vi "test udp++2.vi"() -> ()   [LabVIEW 2017]
uses:
  <vilib>/Platform/TimedLoop/XDataNode/timing_clust.ctl
  <vilib>/Platform/TimedLoop/XDataNode/nitl_modes.ctl
  <vilib>/Platform/TimedLoop/XDataNode/wakeup.ctl
  <vilib>/Platform/TimedLoop/XDataNode/XDataNode.xnode
  <vilib>/Platform/TimedLoop/XDataNode/XDNodeRunTimeDep.lvlib
  UDP++.lvlib
panel:
  in  "stop":bool
  out "sumcheck":dbl[](array[numeric])
  out "Validation send":dbl[](array[numeric])
  in  "Numeric":i32=1000
  out "Array":dbl[](array[numeric])
  out "接收控制指令":dbl[](array[numeric])
  out "wifi_KongZ":bool
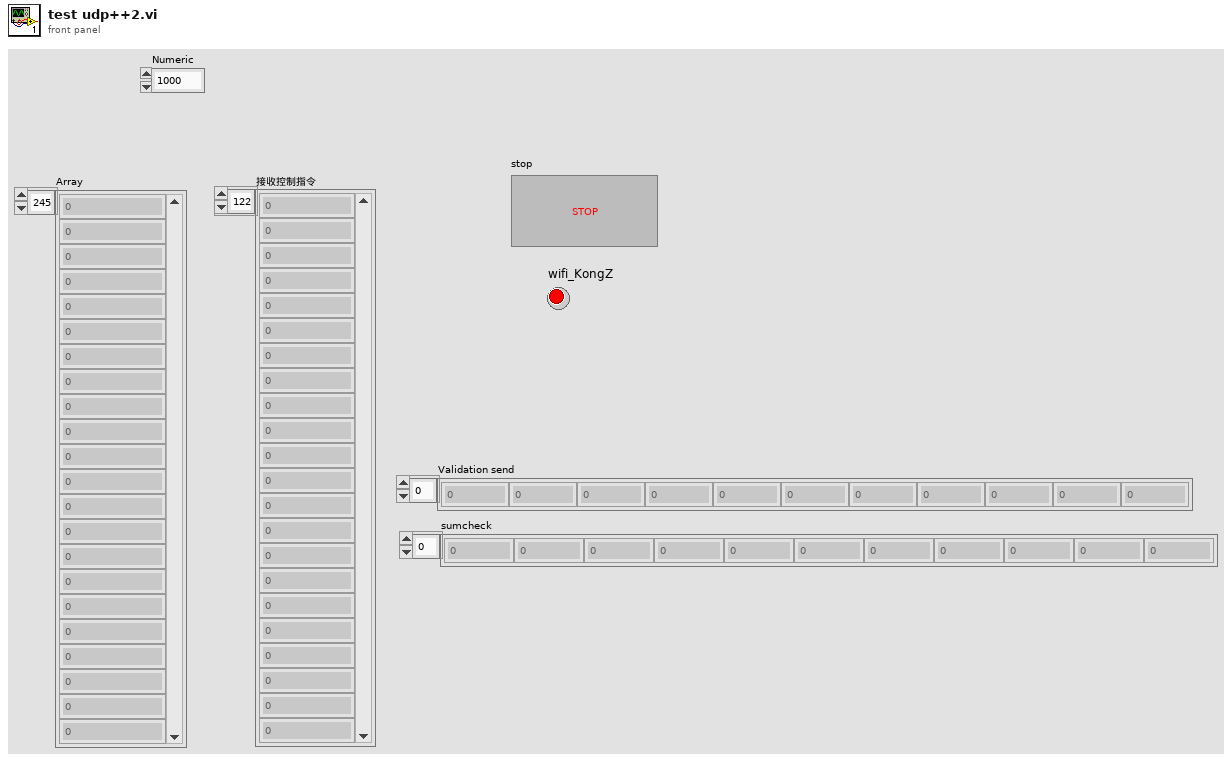
[diagram p1: front panel]
types:
  T1 = cluster{"本地IP":string, "本地端口":u16, "远程IP":string, "远程端口":u16}
  T2 = typedef "XDNodeRunTimeDep.lvlib/timing_clust.ctl" = cluster{"Expected End [f-1]":u64, "Actual End [f-1]":u64, "Finished Late? [f-1]":bool, "Expected End [i-1]":u64, "Actual End [i-1]":u64, "Finished Late? [i-1]":bool, "Expected Start [i]":u64, "Actual Start [i]":u64, "Expected Start [f]":u64, "Actual Start [f]":u64, "Source Name":string, "Structure Name":string, "Period":i64, "Deadline":i64, "Offset":i64, "Start":i64, "Priority":i32, "Timeout":i32, "Mode":T3, "Wakeup Reason":T4, "Error":errorcluster, "Source Type":string, "Secondary Source Type":string, "Global End Time":u64, "Global Start Time":u64, "Frame Duration":u64, "Iteration Duration":u64, "Assigned CPU":i32, "I/O Scan Engine Mode":u32}
  T3 = typedef "XDNodeRunTimeDep.lvlib/nitl_modes.ctl" = enum32{"No Change", "Process missed periods, maintain original phase", "Discard missed periods, maintain original phase", "Process missed periods, ignore original phase", "Discard missed periods, ignore original phase"}
  T4 = typedef "XDNodeRunTimeDep.lvlib/wakeup.ctl" = enum32{"Normal", "Aborted", "Asynchronous wakeup", "Timing source error", "Timed loop error", "Timeout"}
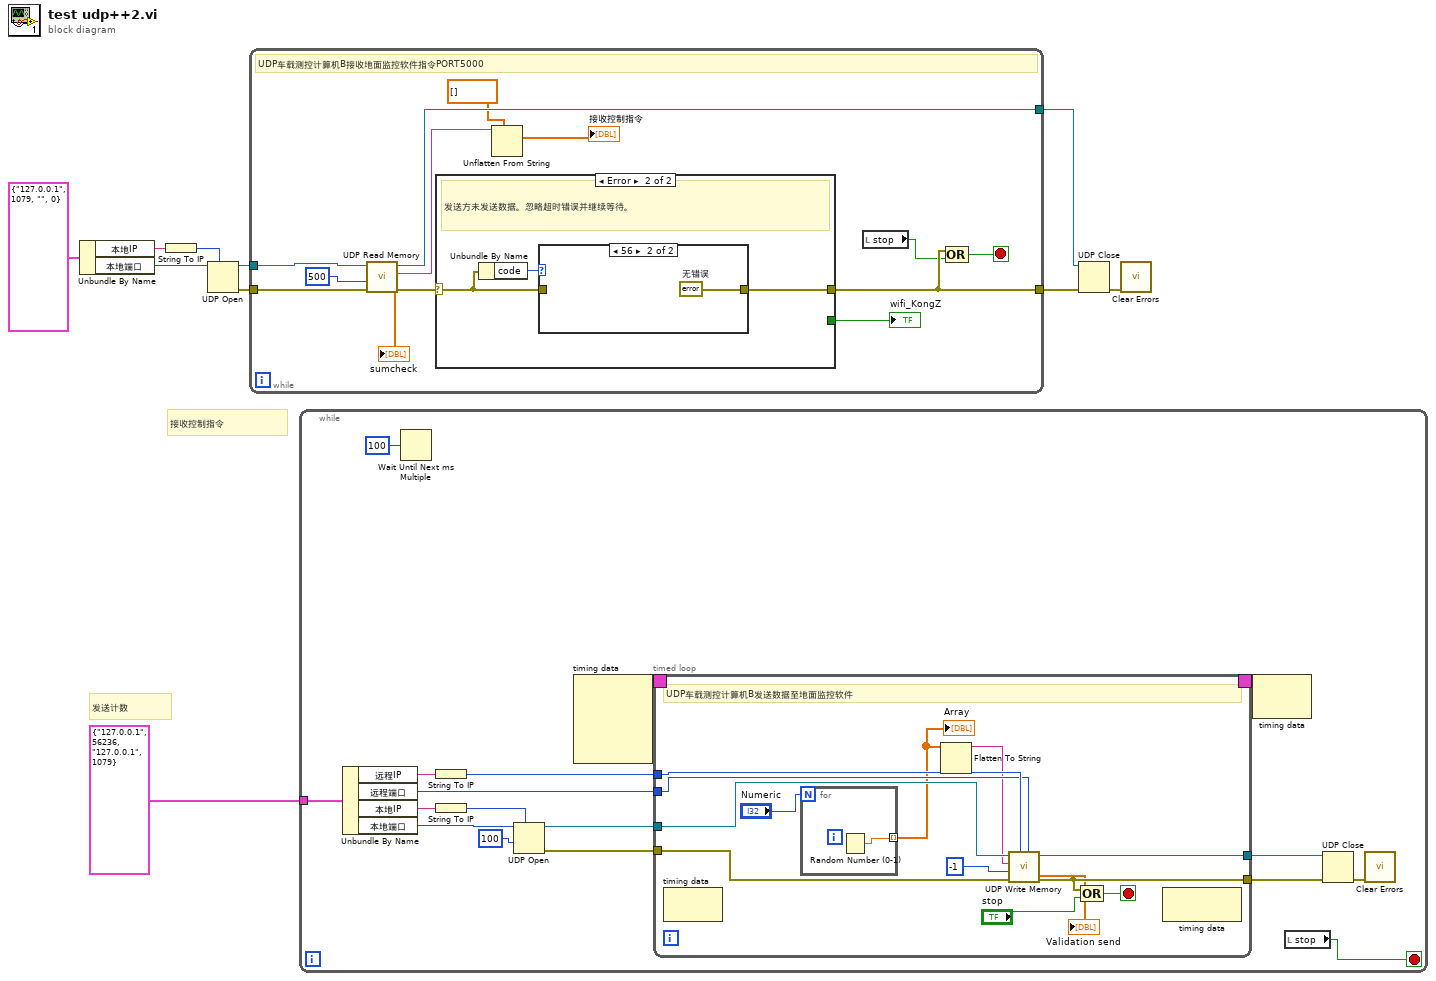
[diagram p0: block diagram]
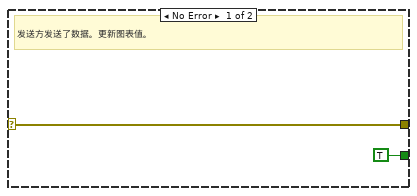
[diagram p2: hidden frame]
diagram:
  # "发送计数"
  # "接收控制指令"
  n1 = Unbundle By Name(T1 {"本地IP"="127.0.0.1", "本地端口"=1079, "远程IP"="", "远程端口"=0} ("UDP配置")) -> ("本地IP"=w3:string, "本地端口"=w2:u16)
  n2 = String To IP(1:w3) -> (0:w10:u32)
  n3 = UDP Open(7:w10, 11:w2) -> (port=w9:refnum<k16>, 0:w8:errorcluster)  [unwired: 3 in, 1 out]
  n4 = while {
    tunnel: w9 -> [w23]
    tunnel: [w21] -> w6
    tunnel: w8 -> [w22]
    tunnel: [w20] -> w7
    stop <- w19 stop-if-true
    # "UDP车载测控计算机B接收地面监控软件指令PORT5000"
    n5 = call "UDP Read Memory.vi"("error in (no error)"=w22, "超时毫秒(25000)"=500, "UDP Network Connection in"=w23) -> ("error out"=w17:errorcluster, "String"=w15:string, "UDP Network Connection out"=w21:refnum<k16>, "checksum"=→"sumcheck":dbl[])  [unwired: 5 in]
    n6 = case shown="Error" w17 {
      selector: w17 -> [w25 w27]
      tunnel: [w25 w26] -> w20
      tunnel: [TRUE ("wifi_KongZ") _] -> w18
      frame No Error {
        # "发送方发送了数据。更新图表值。"
      }
      frame Error {
        # "发送方未发送数据。忽略超时错误并继续等待。"
        n7 = Unbundle By Name(w27) -> ("code"=w28:i32)
        n8 = case shown="56" w28 {
          tunnel: w27 -> [w29 _]
          tunnel: [w29 w30] -> w26
          frame Default {
          }
          frame 56 {
            w30 = errorcluster {"status"=FALSE, "code"=0, "source"=""}  # 无错误
          }
        }
      }
    }
    "wifi_KongZ" <- w18
    n9 = Unflatten From String(type=dbl[] [] ("接收控制指令"), binary string=w15) -> (value=→"接收控制指令":dbl[])  [unwired: 3 in, 2 out]
    n10 = local read "stop"() -> (w11:bool)
    n11 = Compound Arithmetic op=OR ("复合运算")(w20, w11) -> (w19:bool)
  }
  n12 = while {
    tunnel: T1 {"本地IP"="127.0.0.1", "本地端口"=56236, "远程IP"="127.0.0.1", "远程端口"=1079} ("UDP配置") -> [w36]
    stop <- w31 stop-if-true
    n13 = Unbundle By Name(w36) -> ("远程IP"=w33:string, "远程端口"=w32:u16, "本地IP"=w34:string, "本地端口"=w35:u16)
    n14 = Wait Until Next ms Multiple(millisecond multiple=u32 100 ("毫秒倍数")) -> ()  [unwired: 1 out]
    n15 = String To IP(1:w33) -> (0:w41:u32)
    n16 = String To IP(1:w34) -> (0:w43:u32)
    n17 = UDP Open(7:w43, 9:100 ("超时毫秒(25000)"), 11:w35) -> (port=w45:refnum<k16>, 0:w44:errorcluster)  [unwired: 2 in, 1 out]
    n18 = node-c288() -> (w47:T2)  [unwired: 4 in]
    n19 = timed-loop {
      tunnel: [w57] -> w39
      tunnel: w45 -> [w60]
      tunnel: w44 -> [w58]
      tunnel: [w59] -> w38
      tunnel: w32 -> [w53]
      timing: w47 -> [_]
      timing-out: [_] -> w46
      tunnel: w41 -> [w54]
      stop <- w56 stop-if-true
      # "UDP车载测控计算机B发送数据至地面监控软件"
      n20 = node-c288() -> ()  [unwired: 1 in, 1 out]
      n21 = for {
        N: "Numeric" -> [_]
        tunnel: [w61] -> w51 mode=indexing
        n22 = Random Number (0-1)() -> (number: 0 to 1=w61:dbl)
      }
      "Array" <- w51
      n23 = Flatten To String(anything=w51) -> (data string=w50:string)  [unwired: 3 in, 2 out]
      n24 = call "UDP Write Memory.vi"("port or service name"=w53, "address"=w54, "error in (no error)"=w58, "超时毫秒(25000)"=-1, "String"=w50, "UDP Network Connection in"=w60) -> ("error out"=w57:errorcluster, "UDP Network Connection out"=w59:refnum<k16>, "checksum"=→"Validation send":dbl[])  [unwired: 3 in]
      n25 = Compound Arithmetic op=OR ("复合运算")(w57, "stop") -> (w56:bool)
      n26 = node-c288() -> ()  [unwired: 1 in, 1 out]
    }
    n27 = node-c288(w46) -> ()  [unwired: 1 out]
    n28 = local read "stop"() -> (w31:bool)
    n29 = UDP Close(connection ID=w38, 8:w39) -> (error out=w37:errorcluster)  [unwired: 1 out]
    n30 = call <vilib>:"Clear Errors.vi"("error in (no error)"=w37) -> ()  [unwired: 5 in, 2 out]
  }
  n31 = UDP Close(connection ID=w6, 8:w7) -> (error out=w5:errorcluster)  [unwired: 1 out]
  n32 = call <vilib>:"Clear Errors.vi"("error in (no error)"=w5) -> ()  [unwired: 5 in, 2 out]
